vi "Import Dialog.vi"(8 "error in (no error)":errorcluster, 11 "Item Ref in":T1 format="%.0x") -> (0 "error out":errorcluster, 3 "Item Ref out":T1 format="%.0x")   [LabVIEW 2017, in "DSF System Explorer.lvlib"]
uses:
  DSF System Explorer.lvlib
  <vilib>/NI Veristand/Custom Device API/Custom Device Item Ref.ctl
  DSF Core.lvlibp/Typedefs/DSF Engine Framework Configuration.ctl
  DSF Core.lvlibp/Typedefs/DSF Engine Plugin Configuration.ctl
  DSF Core.lvlibp/Typedefs/Core Plugin Configuration.ctl
  DSF Core.lvlibp/Typedefs/DSF Timing Info.ctl
  DSF Core.lvlibp/Typedefs/DSF Settings Info.ctl
  DSF Core.lvlibp/Typedefs/DSF Engine Plugin Thread Configuration.ctl
  DSF Core.lvlibp/Typedefs/Core Thread Configuration.ctl
  DSF Core.lvlibp/Typedefs/DSF Engine Transfer Group Configuration.ctl
  DSF Core.lvlibp/Typedefs/Core Group Configuration.ctl
  DSF Core.lvlibp/Typedefs/DSF Direction.ctl
  DSF Core.lvlibp/Typedefs/DSF Timeout Behavior.ctl
  DSF Core.lvlibp/Typedefs/DSF Engine Transfer Configuration.ctl
  DSF Core.lvlibp/Typedefs/Core Transfer Configuration.ctl
  DSF Core.lvlibp/Typedefs/DSF Engine Channel Configuration.ctl
  DSF Core.lvlibp/Typedefs/Core Channel Configuration.ctl
  DSF Core.lvlibp/Typedefs/DSF Data Type.ctl
  DSF Core.lvlibp/Classes/Configuration Session/Configuration Session.lvclass
  DSF Core.lvlibp
  DSF Core.lvlibp/Classes/Configuration/Core/Plugin/Plugin Configuration.lvclass
  DSF Core.lvlibp/Classes/Configuration/Core/Thread/Thread Configuration.lvclass
  DSF Core.lvlibp/Classes/Configuration/Core/Group/Group Configuration.lvclass
  DSF Core.lvlibp/Classes/Configuration/Core/Transfer/Transfer Configuration.lvclass
  DSF Core.lvlibp/Classes/Configuration/Core/Channel/Channel Configuration.lvclass
  <vilib>/NI Veristand/Custom Device API/Custom Device API.lvlib
panel:
  out "Duration":u32 format="%d ms"
  out "Version":string
  in  "Apply":bool
  in  "Load":bool
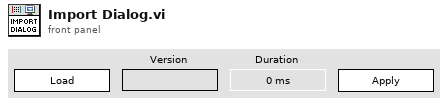
[diagram p1: front panel]
types:
  T1 = typedef "Custom Device API.lvlib/Custom Device Item Ref.ctl" = u64
  T2 = enum8{"Enabled", "Disabled", "Disabled and Grayed Out"}
  T3 = typedef "DSF Core.lvlibp/DSF Engine Framework Configuration.ctl" = cluster{"plugins":T4[]}
  T4 = typedef "DSF Core.lvlibp/DSF Engine Plugin Configuration.ctl" = cluster{"core":T5, "component settings":T7[], "threads":T8[]}
  T5 = typedef "DSF Core.lvlibp/Plugin Configuration.lvclass/Core Plugin Configuration.ctl" = cluster{"name":string, "components":string[], "cycle timing":T6}
  T6 = typedef "DSF Core.lvlibp/DSF Timing Info.ctl" = cluster{"priority":u64, "decimation":u64, "offset":u64}
  T7 = typedef "DSF Core.lvlibp/DSF Settings Info.ctl" = cluster{"component":string, "values":cluster{"key":string, "value":string}[]}
  T8 = typedef "DSF Core.lvlibp/DSF Engine Plugin Thread Configuration.ctl" = cluster{"core":T9, "component settings":T7[], "transfer groups":T10[]}
  T9 = typedef "DSF Core.lvlibp/Thread Configuration.lvclass/Core Thread Configuration.ctl" = cluster{"processor":i32, "priority offset":i16}
  T10 = typedef "DSF Core.lvlibp/DSF Engine Transfer Group Configuration.ctl" = cluster{"core":T11, "component settings":T7[], "transfers":T14[]}
  T11 = typedef "DSF Core.lvlibp/Group Configuration.lvclass/Core Group Configuration.ctl" = cluster{"name":string, "direction":T12, "cycle timing":T6, "timeout behavior":T13, "enable conversion":bool}
  T12 = typedef "DSF Core.lvlibp/DSF Direction.ctl" = enum8{"Tx", "Rx"}
  T13 = typedef "DSF Core.lvlibp/DSF Timeout Behavior.ctl" = enum8{"Increment Late Count", "Throw Error"}
  T14 = typedef "DSF Core.lvlibp/DSF Engine Transfer Configuration.ctl" = cluster{"core":T15, "component settings":T7[], "channels":T16[]}
  T15 = typedef "DSF Core.lvlibp/Transfer Configuration.lvclass/Core Transfer Configuration.ctl" = cluster{"name":string}
  T16 = typedef "DSF Core.lvlibp/DSF Engine Channel Configuration.ctl" = cluster{"core":T17, "component settings":T7[]}
  T17 = typedef "DSF Core.lvlibp/Channel Configuration.lvclass/Core Channel Configuration.ctl" = cluster{"name":string, "units":string, "engine data type":T18, "string data type":T18, "string offset":u64}
  T18 = typedef "DSF Core.lvlibp/DSF Data Type.ctl" = enum8{"Bool", "SGL", "DBL", "I8", "I16", "I32", "I64", "U8", "U16", "U32", "U64"}
  T19 = typedef "DSF Core.lvlibp/DSF Version Info.ctl" = cluster{"major":u32, "minor":u32, "fix":u32, "build":string}
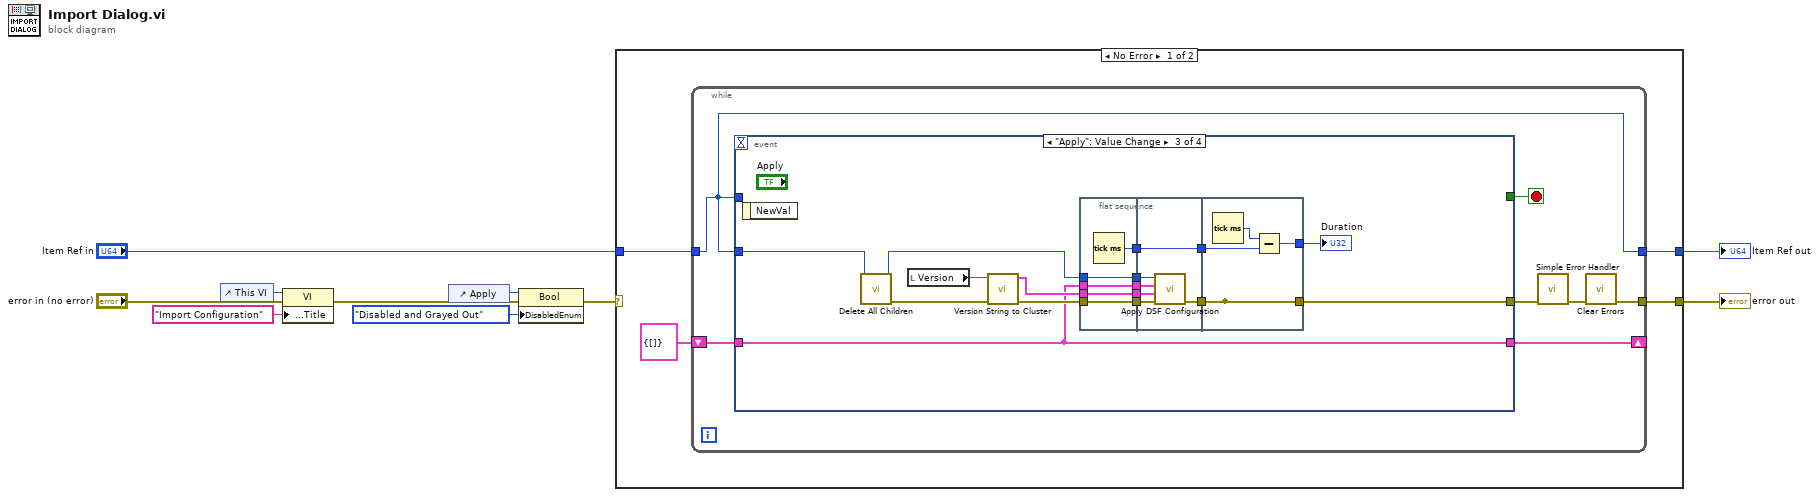
[diagram p0: block diagram]
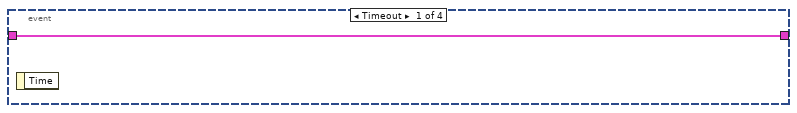
[diagram p2: hidden frame]
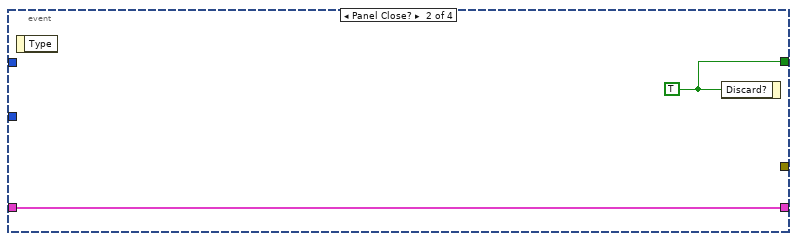
[diagram p3: hidden frame]
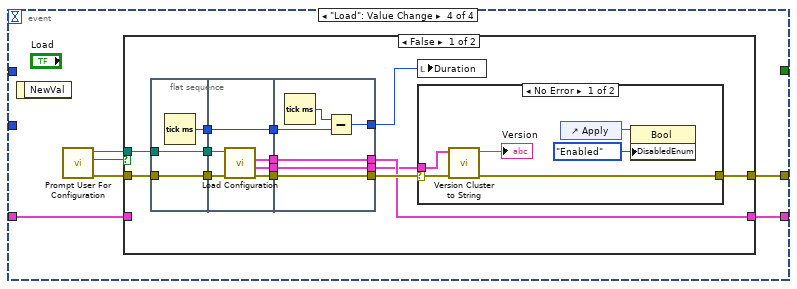
[diagram p4: hidden frame]
diagram:
  n1 = control-ref of="This VI"() -> (w7:refnum<vi>)
  n2 = property class="VI"(reference=w7, error in="error in (no error)", "Front Panel.Title"="Import Configuration" ("Front Panel Window:Title")) -> (error out=w2:errorcluster)  [unwired: 1 out]
  n3 = control-ref of="Apply"() -> (w3:refnum<vi>)
  n4 = property class="Bool"(reference=w3, error in=w2, "DisabledEnum"=T2."Disabled and Grayed Out" ("Disabled")) -> (error out=w1:errorcluster)  [unwired: 1 out]
  n5 = case shown="No Error" w1 {
    selector: w1 -> [_ w100]
    tunnel: [w14 w100] -> w10
    tunnel: "Item Ref in" -> [w13 w101]
    tunnel: [w12 w101] -> w8
    frame No Error {
      n6 = while {
        tunnel: w13 -> [w15]
        tunnel: [w15] -> w12
        shift-right: [w17] -> _
        shift-left: T3 {"plugins"=[]} ("framework configuration") -> [w16]
        tunnel: [w20] -> w14
        stop <- w21 stop-if-true
        n7 = event shown="[2] \"Apply\": Value Change" {
          selector: _ -> [_ _ _ _]
          dyn-events: _ -> [_ _ _ _]
          timeout: _ -> [_ _ _ _]
          tunnel: [_ w23 _ _] -> w21
          tunnel: [_ _ w34 w56] -> w19
          tunnel: w15 -> [_ _ w27 _]
          tunnel: w16 -> [w22 w24 w28 w58]
          tunnel: [w22 w24 w28 w61] -> w17
          tunnel: w15 -> [_ _ _ _]
          event Timeout {
            n8 = event-data() -> ()  [unwired: 1 in, 1 out]
          }
          event Panel Close? {
            w23 = TRUE ("Discard?")
            n9 = event-data() -> ()  [unwired: 1 in, 1 out]
            n10 = event-data("Discard?"=w23) -> ()  [unwired: 1 in, 1 out]
          }
          event "Apply": Value Change {
            n11 = event-data() -> ()  [unwired: 1 in, 1 out]
            n12 = call "Delete All Children.vi"("Item Ref in"=w27) -> ("error out"=w25:errorcluster, "Item Ref out"=w26:T1)  [unwired: 9 in]
            n13 = local read "Version"() -> (w33:string)
            n14 = call "Version String to Cluster.vi"("error in (no error)"=w25, "version string"=w33) -> ("error out"=w32:errorcluster, "version"=w29:T19)  [unwired: 8 in]
            n15 = flat-sequence {
              tunnel: [w45] -> w40
              tunnel: w28 -> [w44]
              tunnel: [w44] -> w36
              tunnel: w26 -> [w43]
              tunnel: [w43] -> w35
              tunnel: w32 -> [w42]
              tunnel: [w42] -> w31
              tunnel: w29 -> [w41]
              tunnel: [w41] -> w30
              tunnel: w40 -> [w51]
              tunnel: [w51] -> w39
              tunnel: [w48] -> w37
              tunnel: w36 -> [w50]
              tunnel: w35 -> [w49]
              tunnel: w31 -> [w47]
              tunnel: w30 -> [w46]
              tunnel: w39 -> [w55]
              tunnel: [w53] -> w38
              tunnel: w37 -> [w52]
              tunnel: [w52] -> _
              tunnel: [w52] -> w34
              frame #0 {
                n16 = Tick Count (ms)() -> (millisecond timer value=w45:u32)
              }
              frame #1 {
                n17 = call "Apply DSF Configuration.vi"("error in (no error)"=w47, "version"=w46, "framework configuration"=w50, "Item Ref in"=w49) -> ("error out"=w48:errorcluster)  [unwired: 7 in]
              }
              frame #2 {
                n18 = Tick Count (ms)() -> (millisecond timer value=w54:u32)
                n19 = Subtract(x=w54, y=w55) -> (x-y=w53:u32)
              }
            }
            "Duration" <- w38
          }
          event "Load": Value Change {
            n20 = event-data() -> ()  [unwired: 1 in, 1 out]
            n21 = call "Prompt User For Configuration.vi"() -> ("error out"=w60:errorcluster, "cancelled"=w57:bool, "selected path"=w59:path)  [unwired: 9 in]
            n22 = case shown="False" w57 {
              tunnel: [w65 w98] -> w56
              tunnel: [w64 w99] -> w61
              tunnel: w60 -> [w75 w98]
              tunnel: w59 -> [w74 _]
              tunnel: w58 -> [_ w99]
              frame False {
                n23 = flat-sequence {
                  tunnel: w74 -> [w84]
                  tunnel: w75 -> [w85]
                  tunnel: [w85] -> w73
                  tunnel: [w84] -> w72
                  tunnel: [w83] -> w68
                  tunnel: w73 -> [w88]
                  tunnel: w72 -> [w87]
                  tunnel: [w91] -> w71
                  tunnel: [w90] -> w70
                  tunnel: [w89] -> w69
                  tunnel: w68 -> [w86]
                  tunnel: [w86] -> w67
                  tunnel: [w95] -> w64
                  tunnel: [w96] -> w66
                  tunnel: [w97] -> w62
                  tunnel: w71 -> [w97]
                  tunnel: w70 -> [w96]
                  tunnel: w69 -> [w95]
                  tunnel: w67 -> [w94]
                  tunnel: [w92] -> w63
                  frame #0 {
                    n24 = Tick Count (ms)() -> (millisecond timer value=w83:u32)
                  }
                  frame #1 {
                    n25 = call "Load Configuration.vi"("error in (no error)"=w88, "configuration file path"=w87) -> ("error out"=w90:errorcluster, "version"=w91:T19, "framework configuration"=w89:T3)  [unwired: 6 in, 1 out]
                  }
                  frame #2 {
                    n26 = Tick Count (ms)() -> (millisecond timer value=w93:u32)
                    n27 = Subtract(x=w93, y=w94) -> (x-y=w92:u32)
                  }
                }
                n28 = local write "Duration"(w63) -> ()
                n29 = case shown="No Error" w66 {
                  selector: w66 -> [w78 w82]
                  tunnel: [w77 w82] -> w65
                  tunnel: w62 -> [w76 _]
                  frame No Error {
                    n30 = call "Version Cluster to String.vi"("error in (no error)"=w78, "version"=w76) -> ("error out"=w77:errorcluster, "version string"=→"Version":string)  [unwired: 8 in]
                    n31 = control-ref of="Apply"() -> (w81:refnum<vi>)
                    n32 = property class="Bool"(reference=w81, "DisabledEnum"=T2."Enabled" ("Disabled")) -> ()  [unwired: 1 in, 2 out]
                  }
                  frame Error {
                  }
                }
              }
              frame True {
              }
            }
          }
        }
        n33 = call <vilib>:"Simple Error Handler.vi"("error in (no error)"=w19) -> ("error out"=w18:errorcluster)  [unwired: 4 in, 4 out]
        n34 = call <vilib>:"Clear Errors.vi"("error in (no error)"=w18) -> ("error out"=w20:errorcluster)  [unwired: 5 in, 1 out]
      }
    }
    frame Error {
    }
  }
  "Item Ref out" <- w8
  "error out" <- w10
